vi "Lab Panel V6.00.vi"() -> ()   [LabVIEW 2017] (continued)
                          tunnel: w3356 -> [_ _ w3369]
                          tunnel: w3355 -> [_ _ w3368]
                          tunnel: w3354 -> [_ _ w3367]
                          tunnel: w3353 -> [_ _ w3366]
                          frame #0 {
                            w3360 = FALSE
                            n1803 = local write "mail control"("END") -> ()
                            n1804 = Bundle(cluster=w3362) -> (w3363:T4)  [unwired: 3 in]
                            n1805 = local write "O/I  LAB05-1"(w3360) -> ()
                            n1806 = local write "RUN LAB05-1"(w3360) -> ()
                            n1807 = local write "run lab05-1"(w3360) -> ()
                            n1808 = local write "DISP LAB05-1"(w3363) -> ()
                          }
                          frame #1 {
                            n1809 = TDMS Close(11:w3364) -> (0:w3365:errorcluster)  [unwired: 1 in, 1 out]
                            n1810 = local write "data file error"(w3365) -> ()
                          }
                          frame #2 {
                            n1811 = stacked-sequence {
                              tunnel: "LAB05-1" -> [w3373 w3379]
                              tunnel: w3370 -> [_ w3378]
                              tunnel: w3369 -> [_ w3377]
                              tunnel: w3368 -> [_ w3376]
                              tunnel: w3367 -> [_ w3375]
                              tunnel: w3366 -> [_ w3374]
                              frame #0 {
                                n1812 = call "sub vi - defrag tdms v1.vi"("panel id"=w3373) -> ("error out"=w3372:errorcluster)  [unwired: 10 in]
                                n1813 = local write "data file error"(w3372) -> ()
                              }
                              frame #1 {
                                n1814 = Bundle("STATUS"=w3378, "OUT SERVER ADDRESS"=w3377, "FROM ACCOUNT"=w3376, "Mail Test File To:"=w3375, "Mail Test Fail"=w3374) -> (w3381:T32)  [unwired: 1 in]
                                n1815 = call "Save data file (pass-fail) v5.vi"("Input Cluster"=w3381, "panel id"=w3379) -> ("network file save error"=w3380:errorcluster)  [unwired: 8 in, 1 out]
                                n1816 = local write "data file error"(w3380) -> ()
                              }
                            }
                          }
                        }
                      }
                    }
                  }
                }
              }
              frame #9 {
                # "LAB05-2"
                n1817 = local read "run lab05-2"() -> (w3386:bool)
                n1818 = case shown="True" w3386 {
                  tunnel: w3385 -> [_ w3391]
                  tunnel: w3384 -> [_ w3390]
                  tunnel: w3383 -> [_ w3389]
                  tunnel: w3382 -> [_ w3388]
                  frame False {
                  }
                  frame True {
                    n1819 = local read "DISP LAB05-2"() -> (w3387:T4)
                    n1820 = Unbundle(w3387) -> ("CYCLE"=w3395:dbl, "STATUS"=w3392:string)  [unwired: 1 out]
                    n1821 = global write "Global display 2.vi" "DISP LAB05-2"(w3387) -> ()
                    n1822 = Not Equal?(x=w3392, y="RUN") -> (x != y?=w3394:bool)
                    n1823 = local read "TDMS LAB05-2"() -> (w3398:refnum<k34>)
                    n1824 = Greater?(x=w3395, y=2.0) -> (0:w3396:bool)
                    n1825 = And(x=w3396, y=w3394) -> (x .and. y?=w3393:bool)
                    n1826 = case shown="True" w3393 {
                      tunnel: w3387 -> [_ w3406]
                      tunnel: w3398 -> [_ w3405]
                      tunnel: w3392 -> [_ w3404]
                      tunnel: w3391 -> [_ w3403]
                      tunnel: w3390 -> [_ w3402]
                      tunnel: w3389 -> [_ w3401]
                      tunnel: w3388 -> [_ w3400]
                      frame False {
                      }
                      frame True {
                        n1827 = stacked-sequence {
                          tunnel: w3406 -> [w3409 _ _]
                          tunnel: w3405 -> [_ w3411 _]
                          tunnel: w3404 -> [_ _ w3417]
                          tunnel: w3403 -> [_ _ w3416]
                          tunnel: w3402 -> [_ _ w3415]
                          tunnel: w3401 -> [_ _ w3414]
                          tunnel: w3400 -> [_ _ w3413]
                          frame #0 {
                            w3407 = FALSE
                            n1828 = local write "mail control"("END") -> ()
                            n1829 = Bundle(cluster=w3409) -> (w3410:T4)  [unwired: 3 in]
                            n1830 = local write "RUN LAB05-2"(w3407) -> ()
                            n1831 = local write "O/I  LAB05-2"(w3407) -> ()
                            n1832 = local write "run lab05-2"(w3407) -> ()
                            n1833 = local write "DISP LAB05-2"(w3410) -> ()
                          }
                          frame #1 {
                            n1834 = TDMS Close(11:w3411) -> (0:w3412:errorcluster)  [unwired: 1 in, 1 out]
                            n1835 = local write "data file error"(w3412) -> ()
                          }
                          frame #2 {
                            n1836 = stacked-sequence {
                              tunnel: "LAB05-2" -> [w3420 w3426]
                              tunnel: w3417 -> [_ w3425]
                              tunnel: w3416 -> [_ w3424]
                              tunnel: w3415 -> [_ w3423]
                              tunnel: w3414 -> [_ w3422]
                              tunnel: w3413 -> [_ w3421]
                              frame #0 {
                                n1837 = call "sub vi - defrag tdms v1.vi"("panel id"=w3420) -> ("error out"=w3419:errorcluster)  [unwired: 10 in]
                                n1838 = local write "data file error"(w3419) -> ()
                              }
                              frame #1 {
                                n1839 = Bundle("STATUS"=w3425, "OUT SERVER ADDRESS"=w3424, "FROM ACCOUNT"=w3423, "Mail Test File To:"=w3422, "Mail Test Fail"=w3421) -> (w3428:T32)  [unwired: 1 in]
                                n1840 = call "Save data file (pass-fail) v5.vi"("Input Cluster"=w3428, "panel id"=w3426) -> ("network file save error"=w3427:errorcluster)  [unwired: 8 in, 1 out]
                                n1841 = local write "data file error"(w3427) -> ()
                              }
                            }
                          }
                        }
                      }
                    }
                  }
                }
              }
            }
            n1842 = global write "Global display 2.vi" "Mail test file to:"(w2935) -> ()
            n1843 = local read "Network Directory"() -> (w2941:path)
            n1844 = global write "Global 1.vi" "Network Drive"(w2941) -> ()
          }
          frame #8 {
            # "disable functions"
            n1845 = stacked-sequence {
              tunnel: w3438 -> [w3452 _ w3509]
              tunnel: w3437 -> [w3447 _ w3508]
              tunnel: w3436 -> [w3446 _ w3507]
              tunnel: w3435 -> [w3444 _ w3506]
              tunnel: w3434 -> [w3445 _ w3505]
              tunnel: w3433 -> [_ w3469 w3504]
              tunnel: w3432 -> [_ w3470 w3503]
              tunnel: w3431 -> [_ w3471 w3502]
              tunnel: w3430 -> [_ w3472 w3501]
              tunnel: w3429 -> [_ w3473 w3500]
              frame #0 {
                n1846 = Select(t=2, s=w3444, f=0) -> (s? t:f=w3440:i32)
                n1847 = Select(t=2, s=w3446, f=0) -> (s? t:f=w3441:i32)
                n1848 = Select(t=2, s=w3445, f=0) -> (s? t:f=w3439:i32)
                n1849 = Select(t=2, s=w3452, f=0) -> (s? t:f=w3443:i32)
                n1850 = Select(t=2, s=w3447, f=0) -> (s? t:f=w3442:i32)
                n1851 = property on="SELECT LAB02-2" class="RadioBtnsControl (strict)"("DisabledEnum"=w3440) -> ()  [unwired: 2 in, 2 out]
                n1852 = property on="SELECT LAB02-1" class="RadioBtnsControl (strict)"("DisabledEnum"=w3441) -> ()  [unwired: 2 in, 2 out]
                n1853 = property on="SELECT LAB03-1" class="RadioBtnsControl (strict)"("DisabledEnum"=w3439) -> ()  [unwired: 2 in, 2 out]
                n1854 = property on="SELECT LAB01-1" class="RadioBtnsControl (strict)"("DisabledEnum"=w3443) -> ()  [unwired: 2 in, 2 out]
                n1855 = property on="SELECT LAB01-2" class="RadioBtnsControl (strict)"("DisabledEnum"=w3442) -> ()  [unwired: 2 in, 2 out]
                n1856 = Not(x=w3452) -> (.not. x?=w3453:bool)
                n1857 = property on="RESULT LAB01-1" class="Bool (strict)"("Visible"=w3453) -> ()  [unwired: 2 in, 2 out]
                n1858 = Not(x=w3447) -> (.not. x?=w3451:bool)
                n1859 = Not(x=w3446) -> (.not. x?=w3450:bool)
                n1860 = Not(x=w3444) -> (.not. x?=w3449:bool)
                n1861 = property on="RESULT LAB01-2" class="Bool (strict)"("Visible"=w3451) -> ()  [unwired: 2 in, 2 out]
                n1862 = Not(x=w3445) -> (.not. x?=w3448:bool)
                n1863 = property on="RESULT LAB02-1" class="Bool (strict)"("Visible"=w3450) -> ()  [unwired: 2 in, 2 out]
                n1864 = property on="RESULT LAB02-2" class="Bool (strict)"("Visible"=w3449) -> ()  [unwired: 2 in, 2 out]
                n1865 = property on="RESULT LAB03-1" class="Bool (strict)"("Visible"=w3448) -> ()  [unwired: 2 in, 2 out]
                n1866 = property on="SET LAB01-1" class="Clust (strict)"("DisabledEnum"=w3443) -> ()  [unwired: 2 in, 2 out]
                n1867 = property on="SET LAB01-2" class="Clust (strict)"("DisabledEnum"=w3442) -> ()  [unwired: 2 in, 2 out]
                n1868 = property on="SET LAB02-1" class="Clust (strict)"("DisabledEnum"=w3441) -> ()  [unwired: 2 in, 2 out]
                n1869 = property on="SET LAB02-2" class="Clust (strict)"("DisabledEnum"=w3440) -> ()  [unwired: 2 in, 2 out]
                n1870 = property on="SET LAB03-1" class="Clust (strict)"("DisabledEnum"=w3439) -> ()  [unwired: 2 in, 2 out]
                n1871 = property on="O/I  LAB01-1" class="Bool (strict)"("DisabledEnum"=w3443) -> ()  [unwired: 2 in, 2 out]
                n1872 = property on="O/I  LAB01-2" class="Bool (strict)"("DisabledEnum"=w3442) -> ()  [unwired: 2 in, 2 out]
                n1873 = property on="O/I  LAB02-1" class="Bool (strict)"("DisabledEnum"=w3441) -> ()  [unwired: 2 in, 2 out]
                n1874 = property on="O/I  LAB02-2" class="Bool (strict)"("DisabledEnum"=w3440) -> ()  [unwired: 2 in, 2 out]
                n1875 = property on="O/I  LAB03-1" class="Bool (strict)"("DisabledEnum"=w3439) -> ()  [unwired: 2 in, 2 out]
              }
              frame #1 {
                n1876 = Select(t=2, s=w3473, f=0) -> (s? t:f=w3464:i32)
                n1877 = Select(t=2, s=w3472, f=0) -> (s? t:f=w3465:i32)
                n1878 = Select(t=2, s=w3469, f=0) -> (s? t:f=w3468:i32)
                n1879 = Select(t=2, s=w3470, f=0) -> (s? t:f=w3467:i32)
                n1880 = Select(t=2, s=w3471, f=0) -> (s? t:f=w3466:i32)
                n1881 = property on="SELECT LAB05-2" class="RadioBtnsControl (strict)"("DisabledEnum"=w3464) -> ()  [unwired: 2 in, 2 out]
                n1882 = property on="SELECT LAB05-1" class="RadioBtnsControl (strict)"("DisabledEnum"=w3465) -> ()  [unwired: 2 in, 2 out]
                n1883 = property on="SELECT LAB03-2" class="RadioBtnsControl (strict)"("DisabledEnum"=w3468) -> ()  [unwired: 2 in, 2 out]
                n1884 = property on="SELECT LAB04-1" class="RadioBtnsControl (strict)"("DisabledEnum"=w3467) -> ()  [unwired: 2 in, 2 out]
                n1885 = property on="SELECT LAB04-2" class="RadioBtnsControl (strict)"("DisabledEnum"=w3466) -> ()  [unwired: 2 in, 2 out]
                n1886 = property on="SET LAB05-2" class="Clust (strict)"("DisabledEnum"=w3464) -> ()  [unwired: 2 in, 2 out]
                n1887 = property on="SET LAB05-1" class="Clust (strict)"("DisabledEnum"=w3465) -> ()  [unwired: 2 in, 2 out]
                n1888 = property on="SET LAB03-2" class="Clust (strict)"("DisabledEnum"=w3468) -> ()  [unwired: 2 in, 2 out]
                n1889 = property on="SET LAB04-1" class="Clust (strict)"("DisabledEnum"=w3467) -> ()  [unwired: 2 in, 2 out]
                n1890 = property on="SET LAB04-2" class="Clust (strict)"("DisabledEnum"=w3466) -> ()  [unwired: 2 in, 2 out]
                n1891 = property on="O/I  LAB05-2" class="Bool (strict)"("DisabledEnum"=w3464) -> ()  [unwired: 2 in, 2 out]
                n1892 = property on="O/I  LAB05-1" class="Bool (strict)"("DisabledEnum"=w3465) -> ()  [unwired: 2 in, 2 out]
                n1893 = property on="O/I  LAB04-1" class="Bool (strict)"("DisabledEnum"=w3467) -> ()  [unwired: 2 in, 2 out]
                n1894 = property on="O/I  LAB04-2" class="Bool (strict)"("DisabledEnum"=w3466) -> ()  [unwired: 2 in, 2 out]
                n1895 = property on="O/I  LAB03-2" class="Bool (strict)"("DisabledEnum"=w3468) -> ()  [unwired: 2 in, 2 out]
                n1896 = Not(x=w3473) -> (.not. x?=w3474:bool)
                n1897 = Not(x=w3472) -> (.not. x?=w3475:bool)
                n1898 = Not(x=w3471) -> (.not. x?=w3476:bool)
                n1899 = property on="RESULT LAB05-2" class="Bool (strict)"("Visible"=w3474) -> ()  [unwired: 2 in, 2 out]
                n1900 = property on="RESULT LAB05-1" class="Bool (strict)"("Visible"=w3475) -> ()  [unwired: 2 in, 2 out]
                n1901 = Not(x=w3470) -> (.not. x?=w3477:bool)
                n1902 = property on="RESULT LAB04-2" class="Bool (strict)"("Visible"=w3476) -> ()  [unwired: 2 in, 2 out]
                n1903 = Not(x=w3469) -> (.not. x?=w3478:bool)
                n1904 = property on="RESULT LAB04-1" class="Bool (strict)"("Visible"=w3477) -> ()  [unwired: 2 in, 2 out]
                n1905 = property on="RESULT LAB03-2" class="Bool (strict)"("Visible"=w3478) -> ()  [unwired: 2 in, 2 out]
              }
              frame #2 {
                # "disable calibrate if any test running"
                n1906 = Or(x=w3501, y=w3500) -> (x .or. y?=w3494:bool)
                n1907 = Or(x=w3503, y=w3502) -> (x .or. y?=w3496:bool)
                n1908 = Or(x=w3507, y=w3506) -> (x .or. y?=w3498:bool)
                n1909 = Or(x=w3505, y=w3504) -> (x .or. y?=w3497:bool)
                n1910 = Or(x=w3509, y=w3508) -> (x .or. y?=w3499:bool)
                n1911 = Or(x=w3497, y=w3496) -> (x .or. y?=w3495:bool)
                n1912 = Or(x=w3499, y=w3498) -> (x .or. y?=w3493:bool)
                n1913 = Or(x=w3495, y=w3494) -> (x .or. y?=w3492:bool)
                n1914 = Or(x=w3493, y=w3492) -> (x .or. y?=w3489:bool)
                "Any Test Running" <- w3489
                n1915 = case shown="False" w3489 {
                  tunnel: [0 2] -> w3491
                  frame False {
                  }
                  frame True {
                  }
                }
                n1916 = property on="JIG TEST" class="Clust (strict)"("DisabledEnum"=w3491) -> ()  [unwired: 2 in, 2 out]
                n1917 = property on="Network Directory" class="Path"("DisabledEnum"=w3491) -> ()  [unwired: 2 in, 2 out]
                n1918 = property on="MAIL SETTINGS" class="Clust (strict)"("DisabledEnum"=w3491) -> ()  [unwired: 2 in, 2 out]
                n1919 = property on="SET (cal)" class="Bool (strict)"("DisabledEnum"=w3491) -> ()  [unwired: 2 in, 2 out]
                n1920 = property on="ADMIN" class="Bool (strict)"("DisabledEnum"=0) -> ()  [unwired: 2 in, 2 out]
              }
            }
          }
          frame #9 {
            # "Note : JIG LAB0X-N   are written to digital I/O in frame 11"
            # "Drive jigs"
            n1921 = stacked-sequence {
              frame #0 {
                # "jig on"
                n1922 = local read "jig cycle"() -> (w3517:dbl)
                n1923 = property on="JIG TEST" class="Clust (strict)"() -> ("DisabledEnum"=w3514:T18)  [unwired: 2 in, 2 out]
                n1924 = Equal?(x=w3514, y=2) -> (x = y?=w3513:bool)
                n1925 = Equal?(x=w3517, y=0) -> (x = y?=w3515:bool)
                n1926 = And(x=w3515, y=w3513) -> (x .and. y?=w3512:bool)
                n1927 = case shown="True" w3512 {
                  frame False {
                  }
                  frame True {
                    n1928 = local read "run lab01-2"() -> (w3527:bool)
                    n1929 = local read "run lab01-1"() -> (w3528:bool)
                    n1930 = local read "run lab02-1"() -> (w3526:bool)
                    n1931 = local read "run lab02-2"() -> (w3525:bool)
                    n1932 = local read "run lab03-1"() -> (w3524:bool)
                    n1933 = local read "run lab03-2"() -> (w3523:bool)
                    n1934 = local read "run lab04-1"() -> (w3522:bool)
                    n1935 = local read "run lab04-2"() -> (w3521:bool)
                    n1936 = local read "run lab05-1"() -> (w3520:bool)
                    n1937 = local read "run lab05-2"() -> (w3519:bool)
                    n1938 = local write "JIG LAB01-2"(w3527) -> ()
                    n1939 = local write "JIG LAB03-2"(w3523) -> ()
                    n1940 = local write "JIG LAB01-1"(w3528) -> ()
                    n1941 = local write "JIG LAB02-1"(w3526) -> ()
                    n1942 = local write "JIG LAB02-2"(w3525) -> ()
                    n1943 = local write "JIG LAB03-1"(w3524) -> ()
                    n1944 = local write "JIG LAB04-1"(w3522) -> ()
                    n1945 = local write "JIG LAB04-2"(w3521) -> ()
                    n1946 = local write "JIG LAB05-1"(w3520) -> ()
                    n1947 = local write "JIG LAB05-2"(w3519) -> ()
                  }
                }
              }
              frame #1 {
                # "jig off"
                n1948 = local read "jig cycle"() -> (w3535:dbl)
                n1949 = local read "on loops"() -> (w3534:dbl)
                n1950 = property on="JIG TEST" class="Clust (strict)"() -> ("DisabledEnum"=w3533:T18)  [unwired: 2 in, 2 out]
                n1951 = Equal?(x=w3533, y=2) -> (x = y?=w3531:bool)
                n1952 = Equal?(x=w3535, y=w3534) -> (x = y?=w3530:bool)
                n1953 = And(x=w3530, y=w3531) -> (x .and. y?=w3529:bool)
                n1954 = case shown="True" w3529 {
                  frame False {
                  }
                  frame True {
                    w3586 = FALSE
                    w3587 = TRUE
                    w3585 = 2
                    n1955 = local read "SELECT LAB05-2"() -> (w3576:T3)
                    n1956 = local read "SELECT LAB04-2"() -> (w3578:T3)
                    n1957 = local read "SELECT LAB04-1"() -> (w3579:T3)
                    n1958 = local read "SELECT LAB05-1"() -> (w3577:T3)
                    n1959 = local read "SELECT LAB03-2"() -> (w3580:T3)
                    n1960 = local read "SELECT LAB02-1"() -> (w3583:T3)
                    n1961 = local read "SELECT LAB03-1"() -> (w3581:T3)
                    n1962 = local read "SELECT LAB02-2"() -> (w3582:T3)
                    n1963 = local read "SELECT LAB01-2"() -> (w3584:T3)
                    n1964 = local read "run lab05-1"() -> (w3546:bool)
                    n1965 = local read "run lab05-2"() -> (w3545:bool)
                    n1966 = local read "run lab04-2"() -> (w3547:bool)
                    n1967 = local read "SELECT LAB01-1"() -> (w3588:T3)
                    n1968 = local read "run lab04-1"() -> (w3548:bool)
                    n1969 = local read "run lab01-1"() -> (w3564:bool)
                    n1970 = local read "run lab01-2"() -> (w3553:bool)
                    n1971 = local read "run lab03-2"() -> (w3549:bool)
                    n1972 = local read "run lab03-1"() -> (w3550:bool)
                    n1973 = local read "run lab02-1"() -> (w3552:bool)
                    n1974 = local read "run lab02-2"() -> (w3551:bool)
                    n1975 = Equal?(x=w3585, y=w3581) -> (x = y?=w3559:bool)
                    n1976 = Equal?(x=w3585, y=w3580) -> (x = y?=w3558:bool)
                    n1977 = Equal?(x=w3585, y=w3579) -> (x = y?=w3557:bool)
                    n1978 = Equal?(x=w3585, y=w3578) -> (x = y?=w3556:bool)
                    n1979 = Equal?(x=w3585, y=w3577) -> (x = y?=w3555:bool)
                    n1980 = Equal?(x=w3585, y=w3576) -> (x = y?=w3554:bool)
                    n1981 = Equal?(x=w3585, y=w3588) -> (x = y?=w3565:bool)
                    n1982 = Equal?(x=w3585, y=w3583) -> (x = y?=w3561:bool)
                    n1983 = Equal?(x=w3585, y=w3582) -> (x = y?=w3560:bool)
                    n1984 = Equal?(x=w3585, y=w3584) -> (x = y?=w3562:bool)
                    n1985 = And(x=w3556, y=w3547) -> (x .and. y?=w3538:bool)
                    n1986 = And(x=w3559, y=w3550) -> (x .and. y?=w3541:bool)
                    n1987 = And(x=w3557, y=w3548) -> (x .and. y?=w3539:bool)
                    n1988 = And(x=w3554, y=w3545) -> (x .and. y?=w3536:bool)
                    n1989 = And(x=w3560, y=w3551) -> (x .and. y?=w3542:bool)
                    n1990 = And(x=w3558, y=w3549) -> (x .and. y?=w3540:bool)
                    n1991 = And(x=w3555, y=w3546) -> (x .and. y?=w3537:bool)
                    n1992 = And(x=w3562, y=w3553) -> (x .and. y?=w3544:bool)
                    n1993 = And(x=w3565, y=w3564) -> (x .and. y?=w3563:bool)
                    n1994 = And(x=w3561, y=w3552) -> (x .and. y?=w3543:bool)
                    n1995 = Select(t=w3587, s=w3563, f=w3586) -> (s? t:f=w3566:bool)
                    n1996 = Select(t=w3587, s=w3544, f=w3586) -> (s? t:f=w3567:bool)
                    n1997 = Select(t=w3587, s=w3543, f=w3586) -> (s? t:f=w3568:bool)
                    n1998 = Select(t=w3587, s=w3542, f=w3586) -> (s? t:f=w3569:bool)
                    n1999 = Select(t=w3587, s=w3541, f=w3586) -> (s? t:f=w3570:bool)
                    n2000 = Select(t=w3587, s=w3540, f=w3586) -> (s? t:f=w3571:bool)
                    n2001 = Select(t=w3587, s=w3539, f=w3586) -> (s? t:f=w3572:bool)
                    n2002 = Select(t=w3587, s=w3538, f=w3586) -> (s? t:f=w3573:bool)
                    n2003 = Select(t=w3587, s=w3537, f=w3586) -> (s? t:f=w3574:bool)
                    n2004 = Select(t=w3587, s=w3536, f=w3586) -> (s? t:f=w3575:bool)
                    n2005 = local write "JIG LAB03-2"(w3571) -> ()
                    n2006 = local write "JIG LAB02-1"(w3568) -> ()
                    n2007 = local write "JIG LAB02-2"(w3569) -> ()
                    n2008 = local write "JIG LAB01-2"(w3567) -> ()
                    n2009 = local write "JIG LAB03-1"(w3570) -> ()
                    n2010 = local write "JIG LAB01-1"(w3566) -> ()
                    n2011 = local write "JIG LAB05-2"(w3575) -> ()
                    n2012 = local write "JIG LAB04-1"(w3572) -> ()
                    n2013 = local write "JIG LAB05-1"(w3574) -> ()
                    n2014 = local write "JIG LAB04-2"(w3573) -> ()
                  }
                }
              }
            }
          }
          frame #10 {
            # "Note : JIG LAB0X-N   are written to digital I/O in frame 11"
            # "enable  jig test output if no test busy"
            n2015 = property on="JIG TEST" class="Clust (strict)"() -> ("DisabledEnum"=w3591:T18)  [unwired: 2 in, 2 out]
            n2016 = Equal?(x=w3591, y=0) -> (x = y?=w3589:bool)
            n2017 = case shown="True" w3589 {
              frame False {
              }
              frame True {
                n2018 = local read "JIG TEST"() -> (w3602:T10)
                n2019 = Unbundle(w3602) -> ("LAB01-1"=w3601:bool, "LAB01-2"=w3600:bool, "LAB02-1"=w3599:bool, "LAB02-2"=w3598:bool, "LAB03-1"=w3597:bool, "LAB03-2"=w3596:bool, "LAB04-1"=w3595:bool, "LAB04-2"=w3594:bool, "LAB05-1"=w3593:bool, "LAB05-2"=w3592:bool)
                n2020 = local write "JIG LAB05-1"(w3593) -> ()
                n2021 = local write "JIG LAB05-2"(w3592) -> ()
                n2022 = local write "JIG LAB04-1"(w3595) -> ()
                n2023 = local write "JIG LAB04-2"(w3594) -> ()
                n2024 = local write "JIG LAB03-2"(w3596) -> ()
                n2025 = local write "JIG LAB01-1"(w3601) -> ()
                n2026 = local write "JIG LAB02-1"(w3599) -> ()
                n2027 = local write "JIG LAB03-1"(w3597) -> ()
                n2028 = local write "JIG LAB01-2"(w3600) -> ()
                n2029 = local write "JIG LAB02-2"(w3598) -> ()
              }
            }
          }
          frame #11 {
            w3606 = FALSE
            # "Drive digital output and RESET  USB and temperature network if required."
            n2030 = global read "Global display 3.vi" "cycle O/F"() -> (w3615:bool)
            n2031 = case shown="False" w3615 {
              tunnel: [w3803 FALSE] -> w3614
              frame False {
                n2032 = local read "Analog error"() -> (w3805:bool)
                n2033 = local read "Reset Measuring"() -> (w3804:bool)
                n2034 = Or(x=w3804, y=w3805) -> (x .or. y?=w3803:bool)
              }
              frame True {
              }
            }
            n2035 = local read "O/I  LAB01-1"() -> (w3633:bool)
            n2036 = local read "JIG LAB01-1"() -> (w3632:bool)
            n2037 = local read "O/I  LAB01-2"() -> (w3631:bool)
            n2038 = local read "JIG LAB01-2"() -> (w3630:bool)
            n2039 = local read "O/I  LAB02-1"() -> (w3629:bool)
            n2040 = local read "JIG LAB02-1"() -> (w3628:bool)
            n2041 = local read "O/I  LAB02-2"() -> (w3627:bool)
            n2042 = local read "JIG LAB02-2"() -> (w3626:bool)
            n2043 = local read "O/I  LAB03-1"() -> (w3625:bool)
            n2044 = local read "JIG LAB03-1"() -> (w3624:bool)
            n2045 = local read "O/I  LAB03-2"() -> (w3623:bool)
            n2046 = local read "JIG LAB03-2"() -> (w3622:bool)
            n2047 = local read "O/I  LAB04-1"() -> (w3621:bool)
            n2048 = local read "JIG LAB04-1"() -> (w3620:bool)
            n2049 = local read "O/I  LAB04-2"() -> (w3612:bool)
            n2050 = local read "JIG LAB04-2"() -> (w3611:bool)
            n2051 = local read "O/I  LAB05-1"() -> (w3610:bool)
            n2052 = local read "JIG LAB05-1"() -> (w3609:bool)
            n2053 = local read "O/I  LAB05-2"() -> (w3608:bool)
            n2054 = local read "JIG LAB05-2"() -> (w3607:bool)
            n2055 = Build Array(w3626, w3625, w3624, w3623, w3622, w3621, w3620) -> (w3618:bool[])
            n2056 = Build Array(w3633, w3632, w3631, w3630, w3629, w3628, w3627) -> (w3619:bool[])
            n2057 = Build Array(w3612, w3611, w3610, w3609, w3608, w3607, w3606, w3606) -> (w3617:bool[])
            n2058 = local read "DAQ Simulate"() -> (w3604:bool)
            n2059 = Not(x=w3615) -> (.not. x?=w3616:bool)
            n2060 = Not(x=w3604) -> (.not. x?=w3603:bool)
            n2061 = Compound Arithmetic op=AND(w3603, w3616, w3614) -> (w3613:bool)
            n2062 = stacked-sequence {
              tunnel: w3619 -> [w3637 w3694]
              tunnel: w3618 -> [w3636 w3693]
              tunnel: w3617 -> [w3635 w3692]
              tunnel: w3604 -> [w3634 w3695]
              tunnel: w3613 -> [_ w3696]
              tunnel: w3605 -> [_ w3691]
              frame #0 {
                # "drive outputs for normal use"
                n2063 = case shown="False" w3634 {
                  tunnel: w3637 -> [w3640 _]
                  tunnel: w3636 -> [w3639 _]
                  tunnel: w3635 -> [w3638 _]
                  frame False {
                    n2064 = disable-structure shown="Enabled" {
                      disable-tunnel: w3640 -> [w3643 w3690]
                      disable-tunnel: w3639 -> [w3642 w3689]
                      disable-tunnel: w3638 -> [w3641 w3688]
                      frame Disabled {
                        n2065 = while {
                          tunnel: w3643 -> [w3654]
                          tunnel: w3642 -> [w3653]
                          tunnel: w3641 -> [w3652]
                          shift-right: [w3650] -> _
                          shift-left: _ -> [w3649]
                          shift-right: [w3646] -> _
                          shift-left: _ -> [w3648]
                          shift-right: [w3645] -> _
                          shift-left: _ -> [w3647]
                          stop <- FALSE continue-if-true
                          n2066 = First Call?() -> (First Call?: T/F=w3644:bool)
                          n2067 = case shown="False" w3644 {
                            tunnel: w3654 -> [w3664 _]
                            tunnel: w3653 -> [w3663 _]
                            tunnel: w3652 -> [w3662 _]
                            tunnel: [w3660 w3685] -> w3650
                            tunnel: w3649 -> [w3659 _]
                            tunnel: w3648 -> [w3658 _]
                            tunnel: w3647 -> [w3657 _]
                            tunnel: [w3656 w3685] -> w3646
                            tunnel: [w3655 w3685] -> w3645
                            frame False {
                              n2068 = for {
                                N: 4 -> [_]
                                tunnel: w3664 -> [w3682]
                                tunnel: w3663 -> [w3672]
                                tunnel: w3662 -> [w3671]
                                shift-right: [w3667] -> w3660
                                shift-left: w3659 -> [w3683]
                                shift-right: [w3666] -> w3656
                                shift-left: w3658 -> [w3673]
                                shift-right: [w3665] -> w3655
                                shift-left: w3657 -> [w3669]
                                i -> [w3681]
                                # "Drive 2 outputs at a time to reduce noise due to switching"
                                n2069 = Add(x=2, y=w3681) -> (x+y=w3670:i32)
                                n2070 = Array Subset(array=w3682, index=w3670, length=2 ("x")) -> (w3678:bool[])
                                n2071 = Array Subset(array=w3671, index=w3670, length=2) -> (w3674:bool[])
                                n2072 = Array Subset(array=w3672, index=w3670, length=2) -> (w3676:bool[])
                                n2073 = Insert Into Array(array=w3683, index=w3670, new element=w3678) -> (w3667:bool[])
                                "USB OUT 0" <- w3667
                                n2074 = Insert Into Array(array=w3669, index=w3670, new element=w3674) -> (w3665:bool[])
                                "USB OUT 2" <- w3665
                                n2075 = Insert Into Array(array=w3673, index=w3670, new element=w3676) -> (w3666:bool[])
                                "USB OUT 1" <- w3666
                                n2076 = call "sub vi - Drive Relays All v6.vi"("Array #2"=w3665, "Array #1"=w3666, "Array #0"=w3667) -> ("error Array"=w3668:errorcluster[])  [unwired: 8 in]
                                n2077 = flat-sequence {
                                tunnel: w3668 -> [_]
                                frame #0 {
                                n2078 = Wait (ms)(milliseconds to wait="DigOutDelay") -> ()  [unwired: 1 out]
                                }
                                }
                              }
                            }
                            frame True {
                              n2079 = Initialize Array(FALSE, 8 ("dimension size")) -> (w3685:bool[])
                            }
                          }
                        }
                      }
                      frame Enabled {
                        n2080 = local write "USB OUT 1"(w3689) -> ()
                        n2081 = local write "USB OUT 0"(w3690) -> ()
                        n2082 = local write "USB OUT 2"(w3688) -> ()
                        n2083 = call "sub vi - Drive Relays All v6.vi"("Array #2"=w3688, "Array #1"=w3689, "Array #0"=w3690) -> ()  [unwired: 8 in, 1 out]
                      }
                    }
                  }
                  frame True {
                  }
                }
              }
              frame #1 {
                # "USB  reset routine"
                n2084 = case shown="True" w3696 {
                  tunnel: w3695 -> [_ w3701]
                  tunnel: w3694 -> [_ w3700]
                  tunnel: w3693 -> [_ w3699]
                  tunnel: w3692 -> [_ w3698]
                  tunnel: w3691 -> [_ w3697]
                  frame False {
                  }
                  frame True {
                    n2085 = stacked-sequence {
                      seq-local: [w3703 _ _ _ _] -> [_ w3710 _ _ _]
                      tunnel: w3701 -> [_ w3714 _ _ _]
                      tunnel: w3700 -> [_ w3713 _ _ _]
                      tunnel: w3699 -> [_ w3712 _ _ _]
                      tunnel: w3698 -> [_ w3711 _ _ _]
                      tunnel: w3697 -> [_ w3709 _ _ _]
                      frame #0 {
                        n2086 = case shown="False" "Auto Reset" {
                          tunnel: [w3706 FALSE] -> w3704
                          frame False {
                            n2087 = Two Button Dialog(message="System reset") -> (T button?=w3706:bool)  [unwired: 2 in]
                          }
                          frame True {
                          }
                        }
                        n2088 = disable-structure shown="Disabled" {
                          frame Disabled {
                            n2089 = local write "Tab Control 2"(5) -> ()
                          }
                          frame Enabled {
                          }
                        }
                        n2090 = Or(x="Auto Reset", y=w3704) -> (x .or. y?=w3703:bool)
                      }
                      frame #1 {
                        n2091 = case shown="True" w3710 {
                          tunnel: w3714 -> [_ w3721]
                          tunnel: w3713 -> [_ w3720]
                          tunnel: w3712 -> [_ w3719]
                          tunnel: w3711 -> [_ w3718]
                          tunnel: w3709 -> [_ w3715]
                          frame False {
                          }
                          frame True {
                            n2092 = stacked-sequence {
                              tunnel: w3721 -> [_ w3740 _]
                              tunnel: bool[] [] -> [w3724 w3739 w3760]
                              tunnel: w3720 -> [_ _ w3759]
                              tunnel: w3719 -> [w3723 _ w3758]
                              tunnel: w3718 -> [w3722 _ w3757]
                              tunnel: 5000 -> [w3725 _ w3756]
                              tunnel: w3715 -> [_ w3738 _]
                              frame #0 {
                                # "switch off test stations for system reset"
                                n2093 = stacked-sequence {
                                tunnel: w3725 -> [w3729 w3733 w3735]
                                tunnel: w3724 -> [w3728 w3732 w3736]
                                tunnel: w3723 -> [w3727 _ _]
                                tunnel: w3722 -> [w3726 w3731 _]
                                frame #0 {
                                # "drive 1st 7 inputs"
                                n2094 = call "sub vi - Drive Relays All v6.vi"("Array #2"=w3726, "Array #1"=w3727, "Array #0"=w3728) -> ()  [unwired: 8 in, 1 out]
                                n2095 = call "Message Display V1.vi"("Message"="Delay off LAB 01-1 to 02-1", "Delay mS"=w3729) -> ()  [unwired: 10 in]
                                }
                                frame #1 {
                                # "drive 2nd 7 inputs"
                                n2096 = call "sub vi - Drive Relays All v6.vi"("Array #2"=w3731, "Array #1"=w3732, "Array #0"=w3732) -> ()  [unwired: 8 in, 1 out]
                                n2097 = call "Message Display V1.vi"("Message"="Delay off LAB 02-2 to 04-1", "Delay mS"=w3733) -> ()  [unwired: 10 in]
                                }
                                frame #2 {
                                # "drive 3rd 7 inputs"
                                n2098 = call "sub vi - Drive Relays All v6.vi"("Array #2"=w3736, "Array #1"=w3736, "Array #0"=w3736) -> ()  [unwired: 8 in, 1 out]
                                n2099 = call "Message Display V1.vi"("Message"="Delay off LAB 04-2 to 05-2", "Delay mS"=w3735) -> ()  [unwired: 10 in]
                                }
                                }
                              }
                              frame #1 {
                                # "reset all usb modules"
                                n2100 = stacked-sequence {
                                tunnel: w3740 -> [_ w3746]
                                tunnel: w3739 -> [w3743 _]
                                tunnel: w3738 -> [_ w3744]
                                frame #0 {
                                n2101 = local write "AI Task"(FALSE) -> ()
                                n2102 = call "sub vi - Drive Relays All v6.vi"("Array #2"=bool[] [FALSE, FALSE, FALSE, FALSE, FALSE, FALSE, TRUE, FALSE], "Array #1"=w3743, "Array #0"=w3743) -> ()  [unwired: 8 in, 1 out]
                                }
                                frame #1 {
                                n2103 = call "Reset Meas v 5.vi"("simulate"=w3746) -> ("Reset Error"=w3745:bool)  [unwired: 10 in]
                                n2104 = case shown="True" w3745 {
                                tunnel: w3744 -> [_ w3748]
                                frame False {
                                "Reset Error" <- FALSE
                                }
                                frame True {
                                n2105 = local read "RATE (Hz)"() -> (w3752:dbl)
                                n2106 = local read "SAMPLES"() -> (w3751:dbl)
                                n2107 = call "sub vi - AI USB4704 (3)  Create Task v4.vi"("Test"=w3748, "Rate Hz"=w3752, "Samples"=w3751) -> ("TASK USB 0"=w3755:i32, "TASK USB 1"=w3754:i32, "TASK USB 2"=w3753:i32, "AI Task Er"=w3749:bool)  [unwired: 5 in, 4 out]
                                n2108 = local write "AI Task"(TRUE) -> ()
                                n2109 = local write "Reset Error"(w3749) -> ()
                                n2110 = local write "AI Task2"(w3753) -> ()
                                n2111 = local write "AI Task1"(w3754) -> ()
                                n2112 = local write "AI Task0"(w3755) -> ()
                                }
                                }
                                }
                                }
                              }
                              frame #2 {
                                # "switch test stations back on after reset"
                                n2113 = stacked-sequence {
                                tunnel: w3760 -> [w3764 w3767 _]
                                tunnel: w3759 -> [w3763 w3769 w3774]
                                tunnel: w3756 -> [w3762 w3765 w3771]
                                tunnel: w3758 -> [_ w3768 w3773]
                                tunnel: w3757 -> [_ _ w3770]
                                frame #0 {
                                # "drive 1st 7 inputs"
                                n2114 = call "sub vi - Drive Relays All v6.vi"("Array #2"=w3764, "Array #1"=w3764, "Array #0"=w3763) -> ()  [unwired: 8 in, 1 out]
                                n2115 = call "Message Display V1.vi"("Message"="Delay on LAB 01-1 to 02-1", "Delay mS"=w3762) -> ()  [unwired: 10 in]
                                }
                                frame #1 {
                                # "drive 1st & 2nd outputs"
                                n2116 = call "sub vi - Drive Relays All v6.vi"("Array #2"=w3767, "Array #1"=w3768, "Array #0"=w3769) -> ()  [unwired: 8 in, 1 out]
                                n2117 = call "Message Display V1.vi"("Message"="Delay on LAB 02-2 to 04-1", "Delay mS"=w3765) -> ()  [unwired: 10 in]
                                }
                                frame #2 {
                                n2118 = call "sub vi - Drive Relays All v6.vi"("Array #2"=w3770, "Array #1"=w3773, "Array #0"=w3774) -> ()  [unwired: 8 in, 1 out]
                                n2119 = call "Message Display V1.vi"("Message"="Delay on LAB 04-2 to 05-2", "Delay mS"=w3771) -> ()  [unwired: 10 in]
                                }
                                }
                              }
                            }
                          }
                        }
                      }
                      frame #2 {
                        w3775 = 0
                        w3776 = FALSE
                        # "set all back to zero"
                        n2120 = local read "Total USB resets"() -> (w3778:dbl)
                        n2121 = local read "Resets Done"() -> (w3780:dbl)
                        n2122 = local write "Reset Measuring"(w3776) -> ()
                        n2123 = local write "Analog error"(w3776) -> ()
                        n2124 = local write "Er USB#2"(w3775) -> ()
                        n2125 = local write "Er USB#0"(w3775) -> ()
                        n2126 = local write "Er USB#1"(w3775) -> ()
                        n2127 = local write "Error USB #0"(w3776) -> ()
                        n2128 = local write "Error USB #1"(w3776) -> ()
                        n2129 = local write "Error USB #2"(w3776) -> ()
                        n2130 = Increment(x=w3778) -> (x+1=w3777:dbl)
                        n2131 = Increment(x=w3780) -> (x+1=→"Resets Done":dbl)
                        n2132 = local write "Total USB resets"(w3777) -> ()
                      }
                      frame #3 {
                        # "save reset value"
                        n2133 = String To Path(string="c:\\crabtree\\Set Up\\") -> (path=w3790:path)
                        n2134 = Build Path(base path=w3790, name or relative path="USB resets.bin") -> (appended path=w3783:path)
                        n2135 = Create Folder(path (use dialog)=w3790) -> (error out=w3782:errorcluster)  [unwired: 2 in, 2 out]
                        n2136 = local read "Total USB resets"() -> (w3781:dbl)
                        n2137 = call <vilib>:"Clear Errors.vi"("error in (no error)"=w3782) -> ()  [unwired: 5 in, 2 out]
                        n2138 = Open/Create/Replace File(file path (use dialog)=w3783, operation (0:open)=T19."replace or create") -> (refnum out=w3788:refnum<file>, error out=w3787:errorcluster)  [unwired: 4 in, 1 out]
                        n2139 = Write to Binary File(file (use dialog)=w3788, data=w3781, error in=w3787) -> (refnum out=w3786:refnum<file>, error out=w3785:errorcluster)  [unwired: 3 in, 1 out]
                        n2140 = Close File(refnum=w3786, error in=w3785) -> (error out=w3784:errorcluster)  [unwired: 1 out]
                        n2141 = local write "data file error"(w3784) -> ()
                      }
                      frame #4 {
                        # "mail reset value"
                        n2142 = local read "MAIL SETTINGS"() -> (w3796:T7)
                        n2143 = local read "Total USB resets"() -> (w3800:dbl)
                        n2144 = Unbundle(w3796) -> ("OUT SERVER ADDRESS"=w3802:string, "FROM ACCOUNT"=w3801:string)  [unwired: 5 out]
                        n2145 = Number To Decimal String(number=w3800) -> (decimal integer string=w3798:string)  [unwired: 1 in]
                        n2146 = Concatenate Strings("Total USB resets: ", w3798) -> (w3797:string)
                        n2147 = call "Lab Send Mail Test.vi"("TO:"="mikewestwood@gmail.com", "subject"=w3797, "from"=w3801, "out going server"=w3802) -> ("error out"=w3795:errorcluster)  [unwired: 11 in]
                        n2148 = Bundle(cluster=w3796, "mail error"=w3795) -> (w3794:T7)  [unwired: 6 in]
                        n2149 = local write "MAIL SETTINGS"(w3794) -> ()
                      }
                    }
                  }
                }
              }
            }
          }
          frame #12 {
            # "if all test panels are off stop analog read"
            n2150 = local read "O/I  LAB03-1"() -> (w3829:bool)
            n2151 = local read "O/I  LAB03-2"() -> (w3828:bool)
            n2152 = local read "O/I  LAB04-1"() -> (w3827:bool)
            n2153 = local read "O/I  LAB04-2"() -> (w3826:bool)
            n2154 = local read "O/I  LAB05-1"() -> (w3825:bool)
            n2155 = local read "O/I  LAB05-2"() -> (w3824:bool)
            n2156 = local read "O/I  LAB02-2"() -> (w3830:bool)
            n2157 = local read "O/I  LAB02-1"() -> (w3831:bool)
            n2158 = local read "O/I  LAB01-2"() -> (w3832:bool)
            n2159 = local read "O/I  LAB01-1"() -> (w3833:bool)
            n2160 = Or(x=w3825, y=w3824) -> (x .or. y?=w3822:bool)
            n2161 = Or(x=w3827, y=w3826) -> (x .or. y?=w3823:bool)
            n2162 = Or(x=w3831, y=w3830) -> (x .or. y?=w3821:bool)
            n2163 = Or(x=w3829, y=w3828) -> (x .or. y?=w3819:bool)
            n2164 = Or(x=w3833, y=w3832) -> (x .or. y?=w3820:bool)
            n2165 = Or(x=w3823, y=w3822) -> (x .or. y?=w3816:bool)
            n2166 = Or(x=w3820, y=w3821) -> (x .or. y?=w3818:bool)
            n2167 = Or(x=w3818, y=w3819) -> (x .or. y?=w3817:bool)
            n2168 = Or(x=w3817, y=w3816) -> (x .or. y?=w3814:bool)
            n2169 = local read "Any Test Running"() -> (w3815:bool)
            n2170 = local read "AI Task"() -> (w3810:bool)
            n2171 = Or(x=w3814, y=w3815) -> (x .or. y?=w3809:bool)
            n2172 = Not(x=w3809) -> (.not. x?=w3813:bool)
            n2173 = And(x=w3813, y=w3810) -> (x .and. y?=w3812:bool)
            n2174 = Not(x=w3810) -> (.not. x?=w3811:bool)
            n2175 = And(x=w3809, y=w3811) -> (x .and. y?=w3808:bool)
            n2176 = case shown="True" w3812 {
              frame False {
              }
              frame True {
                # "close task if no test"
                n2177 = local write "AI Task"(FALSE) -> ()
                n2178 = call "sub vi - AI USB4704 (3)  Close Task v2.vi"() -> ()  [unwired: 16 in]
              }
            }
            n2179 = case shown="True" w3808 {
              tunnel: w3807 -> [_ w3834]
              frame False {
              }
              frame True {
                # "create task for test"
                n2180 = local read "SAMPLES"() -> (w3836:dbl)
                n2181 = local read "RATE (Hz)"() -> (w3835:dbl)
                n2182 = call "sub vi - AI USB4704 (3)  Create Task v4.vi"("Test"=w3834, "Rate Hz"=w3835, "Samples"=w3836) -> ("TASK USB 0"=w3837:i32, "TASK USB 1"=w3838:i32, "TASK USB 2"=w3839:i32)  [unwired: 5 in, 5 out]
                n2183 = local write "AI Task0"(w3837) -> ()
                n2184 = local write "AI Task1"(w3838) -> ()
                n2185 = local write "AI Task2"(w3839) -> ()
                n2186 = local write "AI Task"(TRUE) -> ()
              }
            }
          }
          frame #13 {
            # "get all analog values from USB devices"
            n2187 = local read "on loops"() -> (w3853:dbl)
            n2188 = local read "jig cycle"() -> (w3850:dbl)
            n2189 = Add(x=w3853, y=3) -> (x+y=w3851:dbl)
            n2190 = Equal?(x=w3850, y=3) -> (x = y?=w3848:bool)
            n2191 = Equal?(x=w3850, y=w3851) -> (x = y?=w3849:bool)
            n2192 = Or(x=w3848, y=w3849) -> (x .or. y?=w3847:bool)
            "Process AIs" <- w3847
            n2193 = global write "Global display 3.vi" "cycle O/F"(w3848) -> ()
            n2194 = call "Check for valid PF.vi"("Min V"="Min V", "Init"=TRUE, "Min I"="Min I") -> ("PF Out"=w3842:dbl)  [unwired: 6 in, 2 out]
            n2195 = case shown="True" w3847 {
              tunnel: w3848 -> [_ w3859]
              tunnel: w3846 -> [_ w3856]
              tunnel: w3842 -> [_ _]
              frame False {
              }
              frame True {
                n2196 = local read "DAQ Simulate"() -> (w3862:bool)
                n2197 = case shown="False" w3862 {
                  tunnel: [w3878 dynamicdata[] [] ("array GRAPH")] -> w3868
                  tunnel: [w3877 w3904] -> w3867
                  tunnel: [w3876 w3904] -> w3866
                  tunnel: [w3875 w3904] -> w3865
                  tunnel: [w3874 w3904] -> w3864
                  tunnel: [w3873 w3904] -> w3863
                  tunnel: w3859 -> [_ w3908]
                  tunnel: [w3872 "Ambient Volts"] -> w3858
                  tunnel: [w3871 bool[] []] -> w3857
                  tunnel: w3856 -> [w3870 _]
                  tunnel: [w3869 0.3 ("Analog loop time")] -> w3855
                  frame False {
                    # "analog in"
                    n2198 = case shown="True" w3870 {
                      tunnel: [dynamicdata[] [] ("array GRAPH") w3898] -> w3878
                      tunnel: [w3880 w3897] -> w3877
                      tunnel: [w3880 w3896] -> w3876
                      tunnel: [w3880 w3895] -> w3875
                      tunnel: [w3880 w3894] -> w3874
                      tunnel: [w3880 w3893] -> w3873
                      tunnel: [3 w3892] -> w3872
                      tunnel: [bool[] [] w3891] -> w3871
                      tunnel: [0.0 w3887] -> w3869
                      frame False {
                        w3881 = 0.0
                        # "no test"
                        n2199 = Bundle(w3881, w3881, w3881, w3881, w3881, w3881) -> (w3880:cluster{dbl, dbl, dbl, dbl, dbl, dbl})  [unwired: 1 in]
                      }
                      frame True {
                        # "test on"
                        n2200 = local read "AI data 0"() -> (w3890:waveform(dbl)[])
